vi "Update inventory.vi"(8 "error in (no error)":errorcluster, 9 "Cost":u8 format="$ %.1f", 10 "Name":string, 11 "Paquetes Disonibles in":refnum<class "Paquetes Disonibles.lvclass">) -> (0 "error out":errorcluster, 3 "Paquetes Disonibles out":refnum<class "Paquetes Disonibles.lvclass">)   [LabVIEW 2020, in "Paquetes Disonibles.lvlib" / "Paquetes Disonibles.lvclass"]
uses:
  Paquetes Disonibles.lvclass
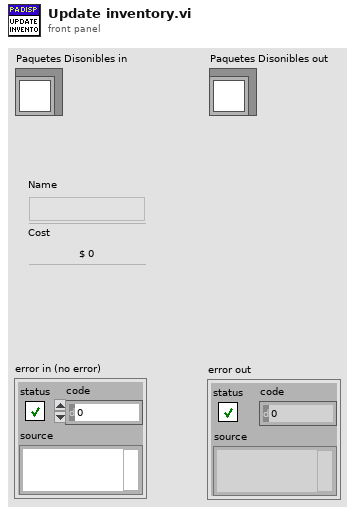
[diagram p1: front panel]
types:
  T1 = cluster{"Products":cluster{"Name":string, "Cost":u8, "Inventory":dbl}, "Products 2":cluster{"Name":string, "Cost":u8, "Inventory":dbl}, "Products 3":cluster{"Name":string, "Cost":u8, "Inventory":dbl}, "Products 4":cluster{"Name":string, "Cost":u8, "Inventory":dbl}, "Products 5":cluster{"Name":string, "Cost":u8, "Inventory":dbl}}
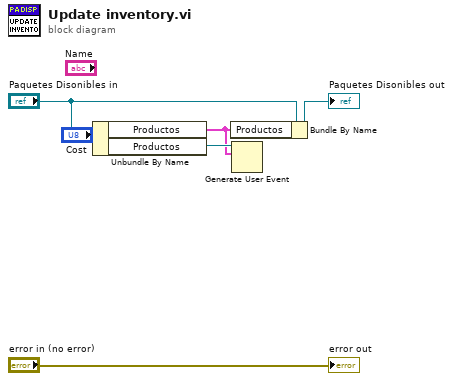
[diagram p0: block diagram]
diagram:
  n1 = Unbundle By Name("Paquetes Disonibles in") -> ("Productos"=w1:T1, "Productos"=w2:refnum<user-event>)
  n2 = Bundle By Name(cluster="Paquetes Disonibles in", "Productos"=w1) -> (→"Paquetes Disonibles out":refnum<class "Paquetes Disonibles.lvclass">)
  n3 = Generate User Event(user event=w2, event data cluster=w1) -> ()  [unwired: 2 in, 2 out]
  "error out" <- "error in (no error)"
